vi "Add Object Parameter - String.vi"(0 "JSON Tree in (JSON Object)":variant, 1 "Name":string, 5 "String":string, 11 "error in (no error)":errorcluster) -> (4 "JSON Tree out (JSON Object)":variant, 15 "error out":errorcluster)   [LabVIEW 2015, in "i3-json.lvlib"]
doc: "Adds a String value to the JSON Tree"
uses:
  i3-json.lvlib
  JSON Types/JSON Type.ctl
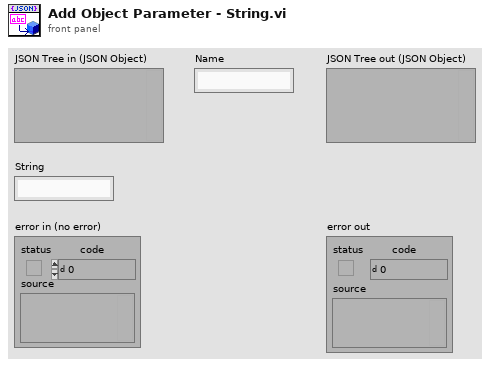
[diagram p1: front panel]
types:
  T1 = typedef "i3-json.lvlib/JSON Type.ctl" = enum8{"JSON Compatible", "JSON Array", "JSON Object", "JSON Null", "Double", "String", "Boolean", "Unknown"}
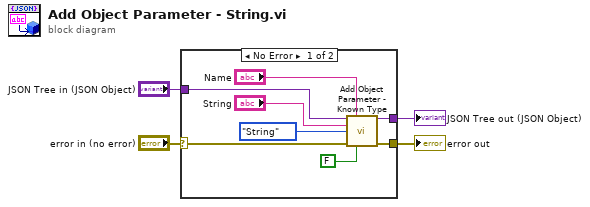
[diagram p0: block diagram]
diagram:
  n1 = case shown="No Error" "error in (no error)" {
    selector: "error in (no error)" -> [w5 w14]
    tunnel: [w12 w14] -> w3
    tunnel: [w11 w13] -> w2
    tunnel: "JSON Tree in (JSON Object)" -> [w10 w13]
    frame No Error {
      n2 = call "Add Object Parameter - Known Type.vi"("JSON Tree in (JSON Object)"=w10, "Name"="Name", "Value"="String", "JSON Type"=JSON_Type."String", "error in (no error)"=w5, "Add Parameter as JSON Tree?"=FALSE) -> ("JSON Tree out (JSON Object)"=w11:variant, "error out"=w12:errorcluster)  [unwired: 8 in]
    }
    frame Error {
    }
  }
  "error out" <- w3
  "JSON Tree out (JSON Object)" <- w2
